vi "load.vi"(8 "error in (no error)":errorcluster, 10 "functional":refnum<user-event>, 11 "interface_dark in":refnum<class "dark.lvclass">=refnum) -> (0 "error out":errorcluster, 3 "interface_dark out":refnum<class "dark.lvclass">)   [LabVIEW 2015, in "example_01.lvlib" / "dark.lvclass"]
uses:
  dark.lvclass
  functional/public/_controls/event_functional_command.ctl
  functional/functional.lvlib
  functional/public/_controls/event_functional.ctl
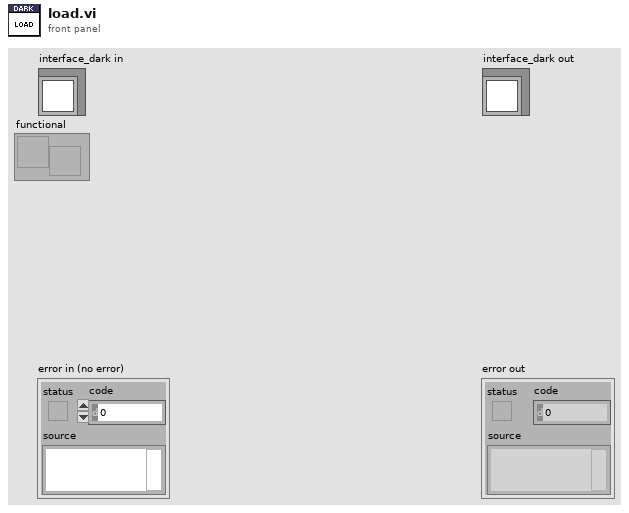
[diagram p1: front panel]
types:
  T1 = enum32{"Invalid", "Standard", "Closed", "Hidden", "Minimized", "Maximized"}
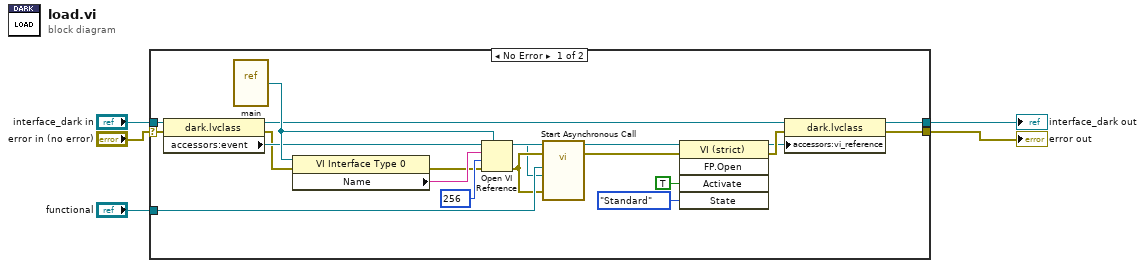
[diagram p0: block diagram]
diagram:
  n1 = case shown="No Error" "error in (no error)" {
    selector: "error in (no error)" -> [w7 w27]
    tunnel: [w10 w27] -> w1
    tunnel: [w14 w26] -> w2
    tunnel: "interface_dark in" -> [w12 w26]
    tunnel: "functional" -> [w25 _]
    frame No Error {
      n2 = property class="dark.lvclass"(reference=w12, error in=w7) -> (reference out=w11:refnum<class "dark.lvclass">, error out=w6:errorcluster, "accessors:event"=w8:refnum<user-event>)
      n3 = vi-ref "main.vi"() -> (w23:refnum<vi>)
      n4 = property class="VI Interface Type 0"(reference=w23, error in=w6) -> (error out=w19:errorcluster, "Name"=w20:string)  [unwired: 1 out]
      n5 = Open VI Reference(type specifier VI Refnum (for type only)=w23, vi path=w20, options=256, error in (no error)=w19) -> (vi reference=w21:refnum<vi>, error out=w22:errorcluster)  [unwired: 2 in]
      n6 = call-by-ref "Start Asynchronous Call"(reference=w21, error in=w22, 8:"error in (no error)"=w22, "event"=w8, "functional"=w25) -> (reference out=w18:refnum<vi>, error out=w17:errorcluster)  [unwired: 8 in, 1 out]
      n7 = invoke class="VI (strict)" method="FP.Open"(reference=w18, error in=w17, "Activate"=TRUE ("Activate?"), "State"=T1."Standard") -> (reference out=w9:refnum<vi>, error out=w13:errorcluster)  [unwired: 1 in, 3 out]
      n8 = property class="dark.lvclass"(reference=w11, error in=w13, "accessors:vi_reference"=w9) -> (reference out=w14:refnum<class "dark.lvclass">, error out=w10:errorcluster)
    }
    frame Error {
    }
  }
  "error out" <- w1
  "interface_dark out" <- w2
